vi "WaitForTime-C.vi"(11 "Params":string[][](array[string])) -> ()   [LabVIEW 2017]
uses:
  Framework/Robot Global Data.vi
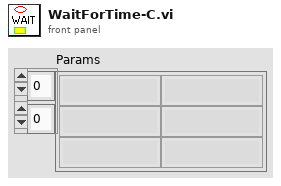
[diagram p1: front panel]
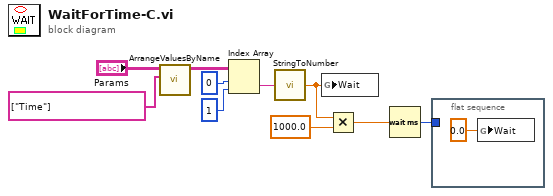
[diagram p0: block diagram]
diagram:
  n1 = call "ArrangeValuesByName.vi"("Names"=string[] ["Time"], "Names/Values in"="Params") -> ("Names/Values Out"=w4:string[][])  [unwired: 9 in]
  n2 = Index Array(array=w4, index (row)=0, index (col)=1) -> (element=w1:string)
  n3 = call "StringToNumber.vi"("String"=w1) -> ("Output"=w9:dbl)
  n4 = global write "Robot Global Data.vi" "Wait"(w9) -> ()
  n5 = Multiply(x=w9, y=1000.0) -> (x*y=w8:dbl)
  n6 = Wait (ms)(milliseconds to wait=w8) -> (millisecond timer value=w7:u32)
  n7 = flat-sequence {
    tunnel: w7 -> [_]
    frame #0 {
      n8 = global write "Robot Global Data.vi" "Wait"(0.0 ("Wait")) -> ()
    }
  }
